vi "ReadLabels.vi"(8 "ErrorIn":errorcluster, 11 "ReferenceIn":refnum<class "VerticalButtonBar.lvclass">) -> (0 "ErrorOut":errorcluster, 2 "Labels":cluster{"Label":string, "Value":string}[](array[cluster]), 3 "ReferenceIn":refnum<class "VerticalButtonBar.lvclass">)   [LabVIEW 2021, in "VerticalButtonBar.lvclass"]
uses:
  VerticalButtonBar.lvclass
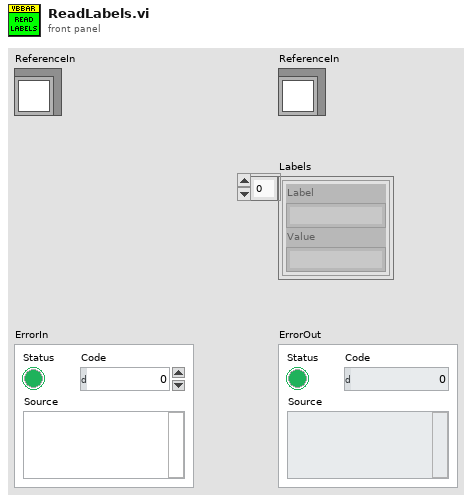
[diagram p1: front panel]
types:
  T1 = typedef "VerticalButtonBar.lvclass/ObjectAttributes.ctl" = cluster{"Interfaces":cluster{"IDockGUI":refnum<class "IDockGUI.lvclass">, "Authorizer":refnum<class "IAuthorization.lvclass">}, "Locals":cluster{"ButtonBar":refnum<class "ButtonCollection.lvclass">, "BaseConfigurationPath":path, "Labels":cluster{"Label":string, "Value":string}[]}, "Persistent":cluster{"ButtonDefinitionFile":string}}
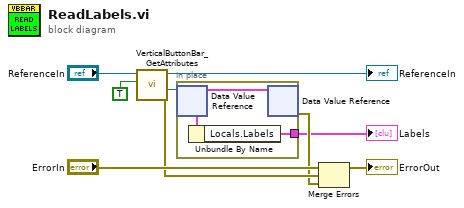
[diagram p0: block diagram]
diagram:
  n1 = call "VerticalButtonBar_GetAttributes.vi"("OnlyGetDvrReference(False)"=TRUE, "ReferenceIn"="ReferenceIn") -> ("ErrorOut"=w8:errorcluster, "DataRef"=w2:refnum<data-value>, "ReferenceOut"=→"ReferenceIn":refnum<class "VerticalButtonBar.lvclass">)  [unwired: 6 in, 1 out]
  n2 = in-place {
    in-place-border: [w11] -> w1
    n3 = in-place-dvr #1(w2) -> (w10:T1)  [unwired: 1 out]
    n4 = Unbundle By Name(w10) -> ("Locals.Labels"=w11:cluster{"Label":string, "Value":string}[])
    n5 = in-place-dvr #1(w10) -> (w6:errorcluster)  [unwired: 1 out]
  }
  "Labels" <- w1
  n6 = Merge Errors("ErrorIn", w8, w6) -> (→"ErrorOut":errorcluster)
